vi "Disconnect.vi"(8 "error in (no error)":errorcluster, 11 "FTP in":refnum<class "FTP.lvclass">) -> (0 "error out":errorcluster, 3 "FTP out":refnum<class "FTP.lvclass">)   [LabVIEW 2013, in "FTP.lvlib" / "FTP.lvclass"]
doc: "This vi will disconnect from the FTP Server, but it won't destroy all of the data that the FTP Toolkit is holding in memory. The FTP.lvclass:Close.vi will both disconnect from the FTP Server and destroy all of the data in memory. The Close.vi will not diconnect from the FTP Server if the server was previously disconnected."
uses:
  FTP.lvclass
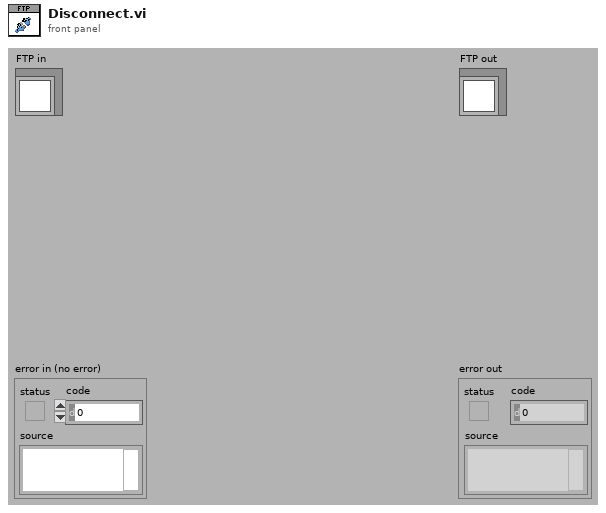
[diagram p1: front panel]
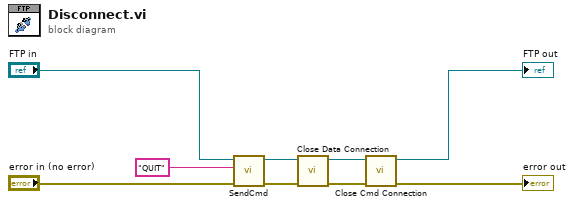
[diagram p0: block diagram]
diagram:
  n1 = call "SendCmd.vi"("error in (no error)"="error in (no error)", "cmd"="QUIT", "FTP in"="FTP in") -> ("error out"=w3:errorcluster, "FTP out"=w4:refnum<class "FTP.lvclass">)  [unwired: 7 in]
  n2 = call "Close Data Connection.vi"("error in (no error)"=w3, "FTP in"=w4) -> ("error out"=w6:errorcluster, "FTP out"=w5:refnum<class "FTP.lvclass">)  [unwired: 8 in]
  n3 = call "Close Cmd Connection.vi"("error in (no error)"=w6, "FTP in"=w5) -> ("error out"=→"error out":errorcluster, "FTP out"=→"FTP out":refnum<class "FTP.lvclass">)  [unwired: 8 in]
